vi "Assert Array Size.vi"(9 "error code":i32=-1, 10 "size":i32, 11 "boolean array":bool[](array[boolean])) -> ()   [LabVIEW 2015, in "niInstr AXI4-Stream Writer v1 FPGA.lvclass"]
doc: "<B>Input Parameters</B>\n\n<B>size</B> is the size of the address space."
uses:
  <instrlib>/_niInstr/CLIP Adapters/v1/FPGA/AXI4-Stream/Writer/niInstr AXI4-Stream Writer v1 FPGA.lvclass
  <instrlib>/_niInstr/Basic Elements/v1/FPGA/niInstr Basic Elements v1 FPGA.lvlib
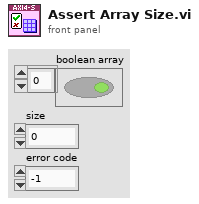
[diagram p1: front panel]
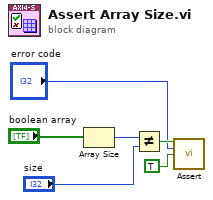
[diagram p0: block diagram]
diagram:
  n1 = Array Size(array="boolean array") -> (size(s)=w6:i32)
  n2 = Not Equal?(x=w6, y="size") -> (x != y?=w5:bool)
  n3 = call <instrlib>:"Assert.vi"("assert"=w5, "error code"="error code", "enable show error"=TRUE) -> ()  [unwired: 13 in]
